vi "Get Scanner Status.vi"(8 "error in (no error)":errorcluster, 11 "Scannable.lvclass in":refnum<class "Scannable.lvclass">) -> (0 "error out":errorcluster, 2 "Status":string, 3 "Scannable.lvclass out":refnum<class "Scannable.lvclass">)   [LabVIEW 2009, in "Scannable.lvclass"]
uses:
  Scannable.lvclass
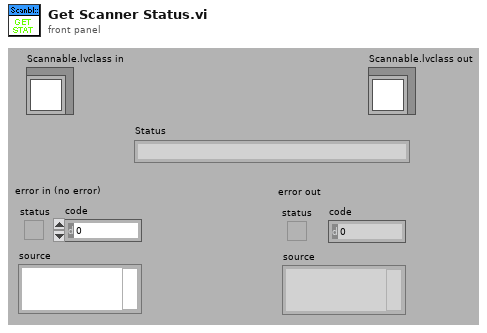
[diagram p1: front panel]
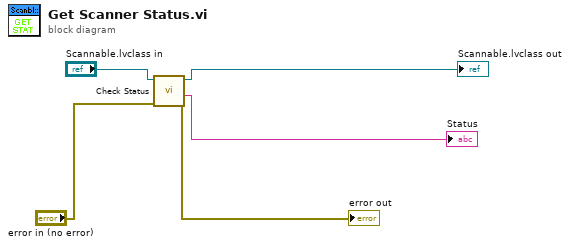
[diagram p0: block diagram]
diagram:
  n1 = call-dynamic "Check Status.vi"("error in (no error)"="error in (no error)", "Instrument in"="Scannable.lvclass in") -> ("error out"=→"error out":errorcluster, "Status"=→"Status":string, "Instrument out"=→"Scannable.lvclass out":refnum<class "Scannable.lvclass">)  [unwired: 6 in, 1 out]
